vi "PythonConfigGlobal.vi"() -> ()   [LabVIEW 2018]
panel:
  in  "python conf":T1
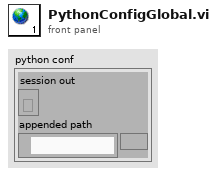
[diagram p1: front panel]
types:
  T1 = cluster{"session out":refnum<k35>, "appended path":path}
diagram:
